vi "RTS Read Configuration Files.vi"(7 "System Number":T1="Select System", 8 "Error In":errorcluster, 11 "Core System Path":path=path "C:/Technology Lab/NI-2010/Trunk/Refrigeration/RTS/Old System") -> (0 "Error Out":errorcluster, 3 "RTS Config Setup Output":T2)   [LabVIEW 2016]
uses:
  Type Definitions/RTS Configuration Setup.ctl
  Type Definitions/RTS Wago Config.ctl
  Type Definitions/RTS APLUS Config.ctl
  Type Definitions/RTS Yokogawa MX Config.ctl
  Type Definitions/RTS Replay Server Control.ctl
  Type Definitions/RTS Server Configuration.ctl
  Type Definitions/RTS Station Settions TCP Comms.ctl
  Type Definitions/RTS Chamber Save Status.ctl
  Type Definitions/RTS Test Pattern.ctl
  Type Definitions/RTS Select System Number.ctl
panel:
  # "W:\\Hooks RTS"
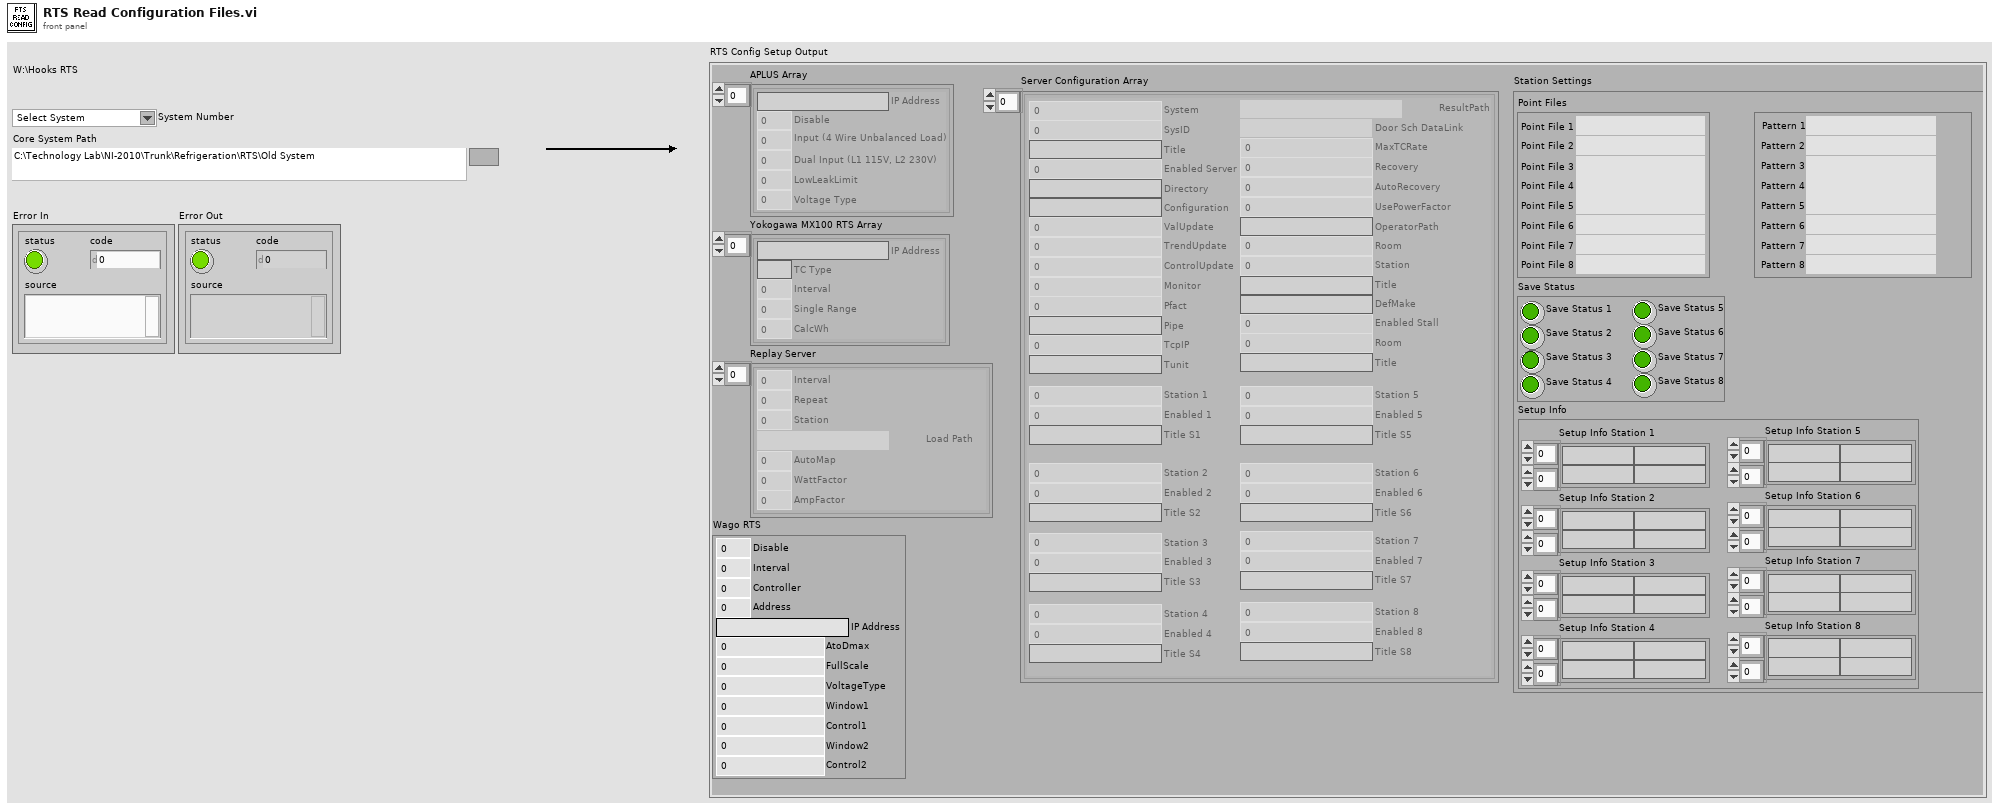
[diagram p1: front panel]
types:
  T1 = typedef "RTS Select System Number.ctl" = string
  T2 = typedef "RTS Configuration Setup.ctl" = cluster{"Wago RTS":T3, "APLUS Array":T4[], "Yokogawa MX100 RTS Array":T5[], "Replay Server":T6[], "Server Configuration Array":T7[], "Station Settings":T8}
  T3 = typedef "RTS Wago Config.ctl" = cluster{"Disable":u16, "Interval":u16, "Controller":u16, "Address":u16, "IP Address":string, "AtoDmax":u16, "FullScale":u16, "VoltageType":u16, "Window1":u16, "Control1":u16, "Window2":u16, "Control2":u16}
  T4 = typedef "RTS APLUS Config.ctl" = cluster{"Disable":u16, "IP Address":string, "Input (4 Wire Unbalanced Load)":u16, "Dual Input (L1 115V, L2 230V)":u16, "LowLeakLimit":dbl, "Voltage Type":u16}
  T5 = typedef "RTS Yokogawa MX Config.ctl" = cluster{"IP Address":string, "TC Type":string, "Interval":u16, "Single Range":u16, "CalcWh":u16}
  T6 = typedef "RTS Replay Server Control.ctl" = cluster{"Interval":i16, "Repeat":u16, "Station":u16, "Load Path":path, "AutoMap":u16, "WattFactor":dbl, "AmpFactor":dbl}
  T7 = typedef "RTS Server Configuration.ctl" = cluster{"System":u16, "SysID":u16, "Title":string, "Enabled Server":u16, "Directory":string, "Configuration":string, "ValUpdate":u16, "TrendUpdate":u16, "ControlUpdate":u16, "Monitor":u16, "Pfact":u16, "Pipe":string, "TcpIP":u16, "Tunit":string, "ResultPath":path, "Door Sch DataLink":path, "MaxTCRate":u16, "Recovery":u16, "AutoRecovery":u16, "UsePowerFactor":u16, "OperatorPath":string, "Room":u16, "Station":u16, "Title":string, "DefMake":string, "Enabled Stall":u16, "Room":u16, "Title":string, "Station 1":u16, "Enabled 1":u16, "Station 2":u16, "Enabled 2":u16, "Station 3":u16, "Enabled 3":u16, "Station 4":u16, "Enabled 4":u16, "Station 5":u16, "Enabled 5":u16, "Station 6":u16, "Enabled 6":u16, "Station 7":u16, "Enabled 7":u16, "Station 8":u16, "Enabled 8":u16, "Title S1":string, "Title S2":string, "Title S3":string, "Title S5":string, "Title S6":string, "Title S7":string, "Title S8":string, "Title S4":string}
  T8 = typedef "RTS Station Settions TCP Comms.ctl" = cluster{"Point Files":cluster{"Point File 1":path, "Point File 2":path, "Point File 3":path, "Point File 4":path, "Point File 5":path, "Point File 6":path, "Point File 7":path, "Point File 8":path}, "Save Status":T9, "Setup Info":cluster{"Setup Info Station 1":string[][], "Setup Info Station 2":string[][], "Setup Info Station 3":string[][], "Setup Info Station 4":string[][], "Setup Info Station 5":string[][], "Setup Info Station 6":string[][], "Setup Info Station 7":string[][], "Setup Info Station 8":string[][]}, "Chamber Test Pattern":T10}
  T9 = typedef "RTS Chamber Save Status.ctl" = cluster{"Save Status 1":bool, "Save Status 2":bool, "Save Status 3":bool, "Save Status 4":bool, "Save Status 5":bool, "Save Status 6":bool, "Save Status 7":bool, "Save Status 8":bool}
  T10 = typedef "RTS Test Pattern.ctl" = cluster{" Pattern 1":path, "Pattern 2":path, "Pattern 3":path, "Pattern 4":path, "Pattern 5":path, "Pattern 6":path, "Pattern 7":path, "Pattern 8":path}
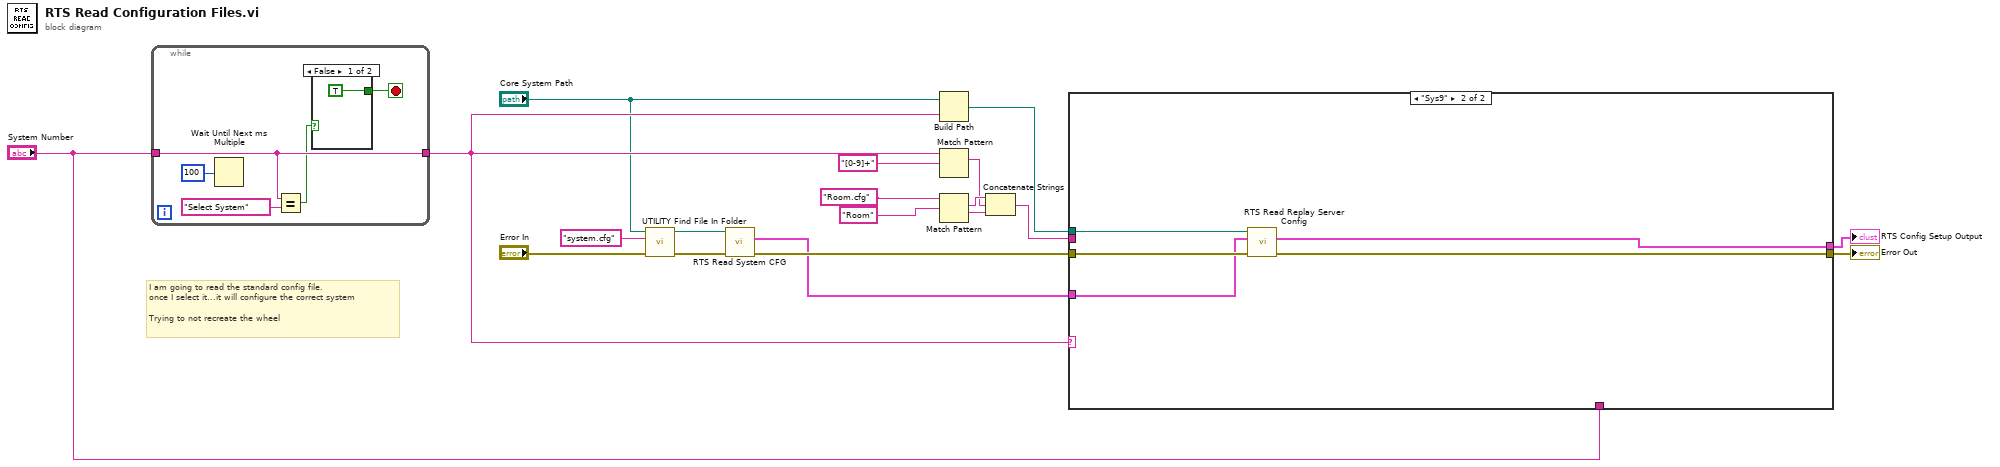
[diagram p0: block diagram]
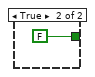
[diagram p2: hidden frame]
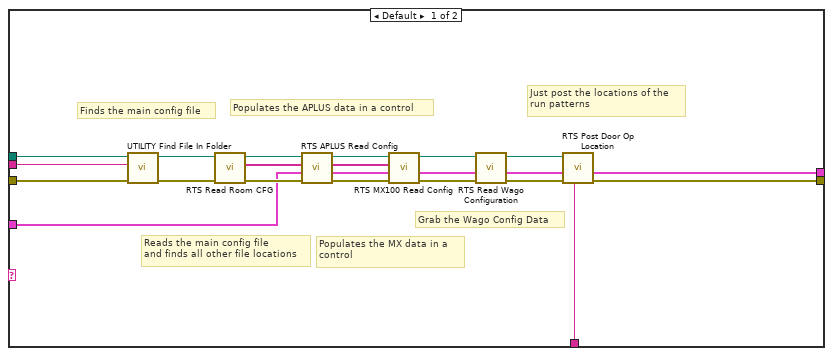
[diagram p3: hidden frame]
diagram:
  # "I am going to read the standard config file.\nonce I select it...it will configure the correct system\n\nTrying to not recreate the wheel"
  n1 = while {
    tunnel: "System Number" -> [w23]
    tunnel: [w23] -> w10
    stop <- w20 stop-if-true
    n2 = Wait Until Next ms Multiple(millisecond multiple=u32 100) -> ()  [unwired: 1 out]
    n3 = Equal?(x=w23, y=T1 "Select System") -> (x = y?=w21:bool)
    n4 = case shown="False" w21 {
      tunnel: [TRUE FALSE] -> w20
      frame False {
      }
      frame True {
      }
    }
  }
  n5 = call "UTILITY Find File In Folder.vi"("Error In"="Error In", "File Name"="system.cfg", "Path"="Core System Path") -> ("Error Out"=w5:errorcluster, "appended path"=w6:path)  [unwired: 7 in]
  n6 = call "RTS Read System CFG.vi"("Error In"=w5, "Room CFG File Path"=w6) -> ("error out"=w4:errorcluster, "Output Configuration"=w3:T2)  [unwired: 7 in, 1 out]
  n7 = Build Path(base path="Core System Path", name or relative path=w10) -> (appended path=w9:path)
  n8 = Match Pattern(string=w10, regular expression="[0-9]+") -> (match substring=w15:T1)  [unwired: 1 in, 3 out]
  n9 = Match Pattern(string="Room.cfg" ("File Name"), regular expression="Room") -> (match substring=w16:string, after substring=w14:string)  [unwired: 1 in, 2 out]
  n10 = Concatenate Strings(w16, w15, w14) -> (w13:string)
  n11 = case shown="\"Sys9\"" w10 {
    tunnel: w9 -> [w47 w52]
    tunnel: w4 -> [w46 w51]
    tunnel: w13 -> [w44 _]
    tunnel: [w32 w50] -> w12
    tunnel: [w30 w53] -> w11
    tunnel: w3 -> [w33 w49]
    tunnel: "System Number" -> [w27 _]
    frame Default {
      # "Just post the locations of the \nrun patterns"
      # "Grab the Wago Config Data"
      # "Populates the MX data in a \ncontrol"
      # "Populates the APLUS data in a control"
      # "Reads the main config file\nand finds all other file locations"
      # "Finds the main config file"
      n12 = call "UTILITY Find File In Folder.vi"("Error In"=w46, "File Name"=w44, "Path"=w47) -> ("Error Out"=w45:errorcluster, "appended path"=w48:path)  [unwired: 7 in]
      n13 = call "RTS Read Room CFG.vi"("Error In"=w45, "Room CFG File Path"=w48) -> ("error out"=w43:errorcluster, "Config Filenames"=w41:string[], "Search File Path"=w42:path)  [unwired: 7 in]
      n14 = call "RTS APLUS Read Config.vi"("Error In"=w43, "RTS Config Setup"=w33, "Config Filenames"=w41, "Search File Path"=w42) -> ("Error Out"=w40:errorcluster, "RTS Config Setup Output"=w36:T2, "Config Filenames Output"=w35:string[], "Search File Path 2"=w38:path)  [unwired: 4 in]
      n15 = call "RTS MX100 Read Config.vi"("Error In"=w40, "RTS Config Setup"=w36, "Config Filenames"=w35, "Search File Path"=w38) -> ("Error Out"=w39:errorcluster, "RTS Config Setup Output"=w34:T2, "Search File Path 2"=w37:path)  [unwired: 4 in, 1 out]
      n16 = call "RTS Read Wago Configuration.vi"("Error In"=w39, "RTS Config Setup Output in"=w34, "Search File Path in"=w37) -> ("error out"=w28:errorcluster, "RTS Config Setup Output out"=w31:T2, "Search File Path Output"=w29:path)  [unwired: 6 in]
      n17 = call "RTS Post Door Op Location.vi"("System Number"=w27, "Error In"=w28, "RTS Config Setup Input"=w31, "Search File Path Output"=w29) -> ("Error Out"=w32:errorcluster, "RTS Config Setup Output"=w30:T2)  [unwired: 6 in]
    }
    frame "Sys9" {
      n18 = call "RTS Read Replay Server Config.vi"("Error In"=w51, "RTS Config Setup Output in"=w49, "Search File Path in"=w52) -> ("Error Out"=w50:errorcluster, "RTS Config Setup Output out"=w53:T2)  [unwired: 7 in]
    }
  }
  "Error Out" <- w12
  "RTS Config Setup Output" <- w11
